vi "Shutdown - on error.vi"(8 "error in (no error)":errorcluster) -> (0 "error out":errorcluster)   [LabVIEW 2026, in "Tests.lvlib"]
doc: "Verifies SRS-LMBR-004: shutdown's flush and close run even when an error is already on the wire. Logs a burst to a file appender, calls Logger.Shutdown with a non-empty incoming error, and asserts every statement was still flushed to the file and the file was closed. Teardown must not skip flush/close on an incoming error, and it must not swallow the caller's error.\n\nImplements LMBR-T-053 -> SRS-004. Assert-level IDs: Test-ID-Assert-Checklist.md."
uses:
  Tests.lvlib
  src/TypeDefs/Severity.ctl
  src/TypeDefs/FileAppenderConfig.ctl
  src/TypeDefs/AppenderConfig.ctl
  src/TypeDefs/Filter.ctl
  src/TypeDefs/FilterMode.ctl
  src/TypeDefs/DropPolicy.ctl
  src/TypeDefs/FileConfig.ctl
  <vilib>/addons/_JKI Toolkits/Caraya/classes/Assert/Assert Error.vi
  <vilib>/addons/_JKI Toolkits/Caraya/classes/Assert/Assert Equal Value_Variant.vi
  <vilib>/addons/_JKI Toolkits/Caraya/classes/Assert/Assert True.vi
  <vilib>/addons/_JKI Toolkits/Caraya/classes/Test/Test.lvclass
  src/Lumberjack.lvlib
  src/Public/Logger.lvclass/Logger.lvclass
  <vilib>/addons/_JKI Toolkits/Caraya/classes/Assert/Assert.lvclass
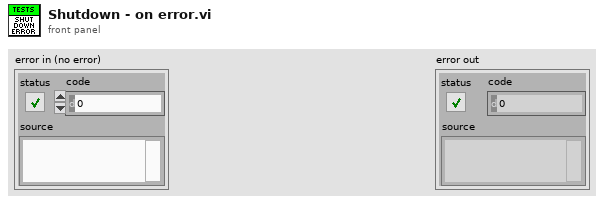
[diagram p1: front panel]
types:
  T1 = typedef "Lumberjack.lvlib/Severity.ctl" = enum16{"OFF", "FATAL", "ERROR", "WARN", "INFO", "DEBUG", "TRACE", "ALL"}
  T2 = typedef "Lumberjack.lvlib/FileAppenderConfig.ctl" = cluster{"common":T3, "file":T7}
  T3 = typedef "Lumberjack.lvlib/AppenderConfig.ctl" = cluster{"id":string, "threshold":T1, "filter":T4, "queueBound":i32, "dropPolicy":T6, "useUTC":bool}
  T4 = typedef "Lumberjack.lvlib/Filter.ctl" = cluster{"mode":T5, "levelMin":T1, "levelMax":T1, "tagPrefix":string}
  T5 = typedef "Lumberjack.lvlib/FilterMode.ctl" = enum16{"Mirror", "Routed"}
  T6 = typedef "Lumberjack.lvlib/DropPolicy.ctl" = enum16{"DropOldest", "DropNewest", "LevelAware"}
  T7 = typedef "Lumberjack.lvlib/FileConfig.ctl" = cluster{"rootFolder":path, "maxFileSize":i64, "maxFileCount":i32, "baseName":string, "extension":string, "delimiter":string, "calendarFolderTree":bool}
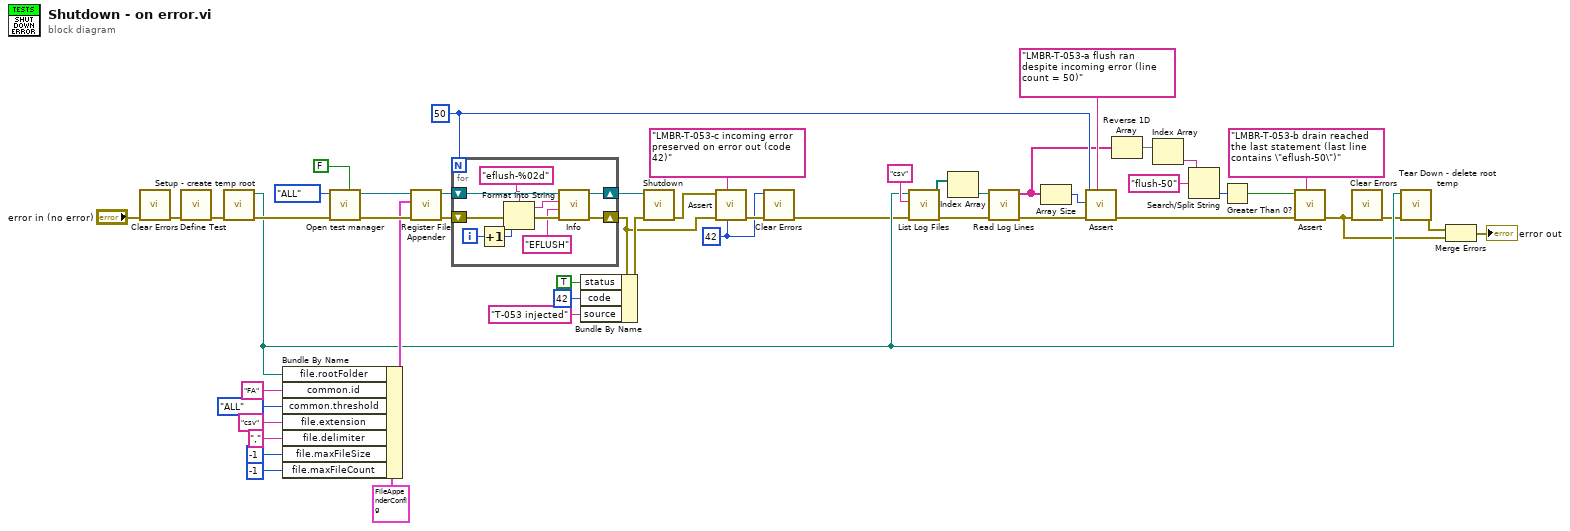
[diagram p0: block diagram]
diagram:
  w1 = 42 ("error code (1)")
  w25 = 50
  n1 = call <vilib>:"Clear Errors.vi"("error in (no error)"="error in (no error)") -> ("error out"=w30:errorcluster)  [unwired: 5 in, 1 out]
  n2 = call <vilib>:"Define Test.vi"("error in (no error)"=w30) -> ("error out"=w49:errorcluster)  [unwired: 9 in, 1 out]
  n3 = call "Setup - create temp root.vi"("error in (no error)"=w49) -> ("error out"=w34:errorcluster, "tempRoot"=w7:path)  [unwired: 9 in]
  n4 = Bundle By Name(cluster=T2 {"common"={"id"="", "threshold"=enum."INFO", "filter"={"mode"=enum."Mirror", "levelMin"=enum."INFO", "levelMax"=enum."INFO", "tagPrefix"=""}, "queueBound"=0, "dropPolicy"=enum."DropOldest", "useUTC"=FALSE}, "file"={"rootFolder"=path "", "maxFileSize"=0, "maxFileCount"=0, "baseName"="", "extension"="", "delimiter"="", "calendarFolderTree"=FALSE}} ("FileAppenderConfig"), "file.rootFolder"=w7, "common.id"="FA", "common.threshold"=Severity."ALL", "file.extension"="csv", "file.delimiter"=",", "file.maxFileSize"=i64 -1, "file.maxFileCount"=-1) -> (w43:T2)
  n5 = call "Open test manager.vi"("enableDefaultFile"=FALSE, "error in (no error)"=w34, "globalThreshold"=Severity."ALL") -> ("error out"=w47:errorcluster, "Logger out"=w42:refnum<class "Logger.lvclass">)  [unwired: 7 in]
  n6 = call "Register File Appender.vi"("error in (no error)"=w47, "FileAppenderConfig"=w43, "Logger in"=w42) -> ("error out"=w46:errorcluster, "Logger out"=w41:refnum<class "Logger.lvclass">)  [unwired: 6 in, 1 out]
  n7 = for {
    N: w25 -> [_]
    shift-right: [w59] -> w9
    shift-left: w46 -> [w57]
    shift-right: [w58] -> w17
    shift-left: w41 -> [w60]
    i -> [w54]
    n8 = Increment(x=w54) -> (x+1=w53:i32)
    n9 = Format Into String(format string="eflush-%02d" ("sourceTag"), error in=w57, w53) -> (resulting string=w52:string, error out=w56:errorcluster)  [unwired: 1 in]
    n10 = call "Info.vi"("error in (no error)"=w56, "sourceTag"="EFLUSH", "message"=w52, "Logger in"=w60) -> ("error out"=w59:errorcluster, "Logger out"=w58:refnum<class "Logger.lvclass">)  [unwired: 6 in]
  }
  n11 = Bundle By Name(cluster=w9, "status"=TRUE, "code"=42, "source"="T-053 injected") -> (w16:errorcluster)
  n12 = call "Shutdown.vi"("error in (no error)"=w16, "Logger in"=w17) -> ("error out"=w10:errorcluster)  [unwired: 9 in]
  n13 = call-poly <vilib>:"Assert.vi"("error code (1)"=w1, "Label"="LMBR-T-053-c incoming error preserved on error out (code 42)", "error in (no error)"=w9, "Error?"=w10) -> ("error out"=w3:errorcluster)  [unwired: 6 in, 1 out]
  n14 = call <vilib>:"Clear Errors.vi"("error in (no error)"=w3, "specific error code to clear (0: all)"=w1) -> ("error out"=w2:errorcluster)  [unwired: 4 in, 1 out]
  n15 = call "List Log Files.vi"("error in (no error)"=w2, "extension"="csv", "rootFolder"=w7) -> ("error out"=w29:errorcluster, "filePaths"=w39:path[])  [unwired: 6 in, 1 out]
  n16 = Index Array(array=w39) -> (element=w32:path)  [unwired: 1 in]
  n17 = call "Read Log Lines.vi"("error in (no error)"=w29, "filePath"=w32) -> ("error out"=w27:errorcluster, "lines"=w21:string[])  [unwired: 8 in]
  n18 = Array Size(array=w21) -> (size(s)=w26:i32)
  n19 = call-poly <vilib>:"Assert.vi"("Label"="LMBR-T-053-a flush ran despite incoming error (line count = 50)", "error in (no error)"=w27, "Actual"=w26, "Expected"=w25) -> ("error out"=w12:errorcluster)  [unwired: 6 in, 1 out]
  n20 = Reverse 1D Array(array=w21) -> (reversed array=w20:string[])
  n21 = Index Array(array=w20) -> (element=w23:string)  [unwired: 1 in]
  n22 = Search/Split String(string=w23, search string/char (-)="flush-50") -> (offset of match=w19:i32)  [unwired: 1 in, 2 out]
  n23 = Greater Than 0?(x=w19) -> (x > 0?=w18:bool)
  n24 = call-poly <vilib>:"Assert.vi"("Label"="LMBR-T-053-b drain reached the last statement (last line contains \"eflush-50\")", "error in (no error)"=w12, "True?"=w18) -> ("error out"=w5:errorcluster)  [unwired: 7 in, 1 out]
  n25 = call <vilib>:"Clear Errors.vi"("error in (no error)"=w5) -> ("error out"=w4:errorcluster)  [unwired: 5 in, 1 out]
  n26 = call "Tear Down - delete root temp.vi"("error in (no error)"=w4, "tempRoot"=w7) -> ("error out"=w8:errorcluster)  [unwired: 9 in]
  n27 = Merge Errors(w8, w5) -> (→"error out":errorcluster)
